vi "close.vi"(8 "error in (no error)":errorcluster, 11 "CSVTestLog in":refnum<class "CSVTestLog.lvclass">) -> (0 "error out":errorcluster, 3 "CSVTestLog out":refnum<class "CSVTestLog.lvclass">)   [LabVIEW 2015, in "CSVTestLog.lvclass"]
uses:
  CSVTestLog.lvclass
  CSVTestLog.lvclass/CSVTestLog.ctl
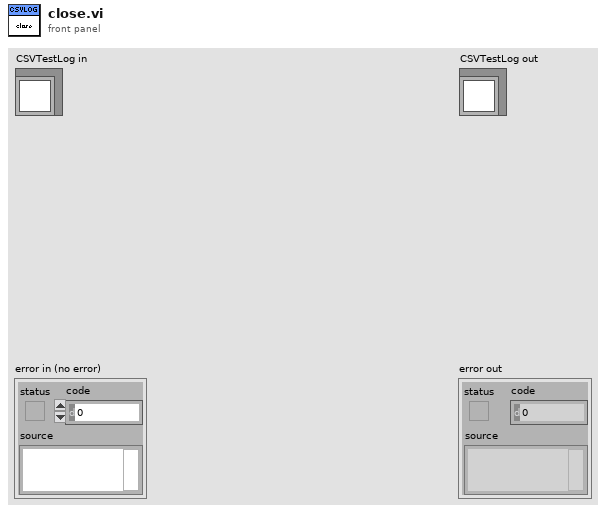
[diagram p1: front panel]
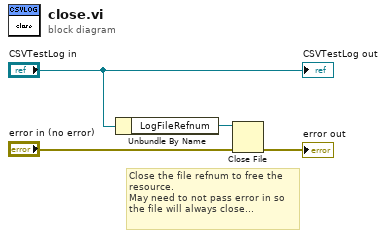
[diagram p0: block diagram]
diagram:
  # "Close the file refnum to free the\nresource.\nMay need to not pass error in so\nthe file will always close..."
  n1 = Unbundle By Name("CSVTestLog in") -> ("LogFileRefnum"=w1:refnum<file>)
  n2 = Close File(refnum=w1, error in="error in (no error)") -> (error out=→"error out":errorcluster)  [unwired: 1 out]
  "CSVTestLog out" <- "CSVTestLog in"
